vi "Act 20.vi"() -> ()   [LabVIEW 2010]
uses:
  act/lv_07/lv_07.lvlib
panel:
  in  "Cc":dbl
  in  "T":dbl
  out "Ccpc init":dbl
  out "T init":dbl
  in  "Ccpc":dbl
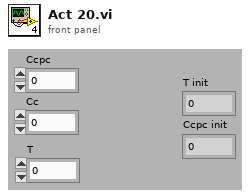
[diagram p1: front panel]
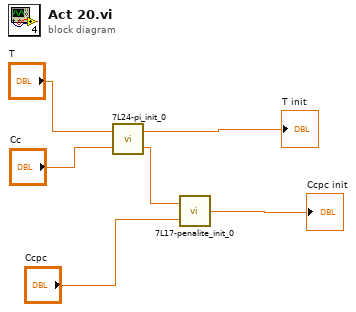
[diagram p0: block diagram]
diagram:
  n1 = call "7L24-pi_init_0.vi"("Cc"="Cc", "T"="T") -> ("Cc init"=w5:dbl, "T init"=→"T init":dbl)
  n2 = call "7L17-penalite_init_0.vi"("Ccpc"="Ccpc", "Cc"=w5) -> ("Ccpc init"=→"Ccpc init":dbl)
